vi "SPI Config Pane.vi"(6 "_SubPanelMessages":refnum<notifier>, 9 "_myEmbeddedToFrameEvent":T9, 10 "_myEmbedded.Exit":refnum<user-event>, 11 "_Property Bundle":cluster{"Name":string, "Value":variant}[](array[cluster])) -> (1 "_Connection Informations":T1, 2 "_Scripter Input":T11)   [LabVIEW 2021]
doc: "Writes data to or reads data from a serial peripheral interface (SPI) slave device."
uses:
  <vilib>/myRIO/Common/Express VI Framework/xctls/myRIO Channel Name/myRIO Channel Name.xctl
  <vilib>/myRIO/Common/Instrument Driver Framework/myRIO v1.0/SPI/typedefs/SPI Frame Length.ctl
  <vilib>/myRIO/Common/Instrument Driver Framework/myRIO v1.0/SPI/typedefs/SPI Clock Phase.ctl
  <vilib>/myRIO/Common/Instrument Driver Framework/myRIO v1.0/SPI/typedefs/SPI Clock Polarity.ctl
  <vilib>/myRIO/Common/Instrument Driver Framework/myRIO v1.0/SPI/typedefs/SPI Data Direction.ctl
  <vilib>/myRIO/Common/Express VI Framework/typedefs/Config Pane to Framework Ref.ctl
  <vilib>/myRIO/Common/Express VI Framework/typedefs/Data Validate Ref.ctl
  <vilib>/myRIO/Common/Express VI Framework/typedefs/Scripter Input.ctl
  <vilib>/myRIO/Common/Express VI Framework/typedefs/WireThrough Terminal Names.ctl
  <vilib>/myRIO/Common/Express VI Framework/typedefs/Instrument Driver Method Descriptor Array.ctl
  <vilib>/myRIO/Common/Express VI Framework/typedefs/Instrument Driver Method Descriptor.ctl
  <vilib>/myRIO/Common/Express VI Framework/typedefs/Sub Panel Messages.ctl
  <vilib>/myRIO/Common/Express VI Framework/typedefs/Connection Informations.ctl
  <vilib>/myRIO/Common/Instrument Driver Framework/Utilities/typedefs/Channel Types.ctl
  <vilib>/myRIO/Instrument Drivers/Onboard IO/SPI/typedefs/SPI User Configuration.ctl
  <vilib>/myRIO/Common/Express VI Framework/vis/Express VI Framework Strings Global.vi
  <vilib>/myRIO/Instrument Drivers/Onboard IO/SPI/SPI.lvlib
panel:
  in  "Channel:":u16(xcontrol)
  out "_learnMoreFrequency":string="Detailed information about valid frequencies for this Express VI.\nLearn more"
  in  "_Validate":bool
  in  "Frequency":dbl=1.0 caption="Frequency:" min=0.0 max=4000000.0
  in  "Frequency Unit":enum16{"Hz", "KHz", "MHz"}(ring)=enum."MHz"
  in  "Mode":enum32{"Write", "Read", "Write/Read"}(radio) caption="Mode:"
  in  "Frame length:":T2=8 min=4 max=16
  in  "Data direction:":T3
  in  "Clock polarity:":T4
  in  "Clock phase:":T5
  out "-Channel Details:":string caption="Connections:"
  in  "_Default Alias String":string
  in  "_VI Default Name (Edit and make value default)":string="SPI"
  in  "Name:":string caption="Node name:"
  in  "_WireThrough Info (Edit and make value default)":T6={"WireThrough Top In"="SPI Ref In", "WireThrough Bottom In"="error in (no error)", "WireThrough Top Out"="SPI Ref Out", "WireThrough Bottom Out"="error out"}
  in  "_Template Array (Edit and make value default)":T7=[{"Function Name"="Smart Open", "VI Path"=path "<vilib>/myRIO/Instrument Drivers/Onboard IO/SPI/vis", "Script"=TRUE, "Inputs"=[{"name"="Channel Name", "value"=variant, "Config Pane Only"=TRUE, "Build Array"=FALSE, "Bundle Cluster"=FALSE, "Show Term"=FALSE, "alias"=[], "Required Input"=FALSE}], "Outputs"=[], "VI Class"=enum."Open", "Controls Refs[]"=[], "Inline"=FALSE}, {"Function Name"="Open", "VI Path"=path "<vilib>/myRIO/Instrument Drivers/Onboard IO/SPI/vis", "Script"=FALSE, "Inputs"=[{"name"="Channel Name", "value"=variant, "Config Pane Only"=TRUE, "Build Array"=FALSE, "Bundle Cluster"=FALSE, "Show Term"=FALSE, "alias"=[], "Required Input"=FALSE}], "Outputs"=[], "VI Class"=enum."Open", "Controls Refs[]"=[], "Inline"=FALSE}, {"Function Name"="Configure", "VI Path"=path "<vilib>/myRIO/Instrument Drivers/Onboard IO/SPI/vis", "Script"=TRUE, "Inputs"=[{"name"="SPI User Configuration", "value"=variant, "Config Pane Only"=TRUE, "Build Array"=FALSE, "Bundle Cluster"=FALSE, "Show Term"=FALSE, "alias"=[], "Required Input"=FALSE}], "Outputs"=[], "VI Class"=enum."Configure", "Controls Refs[]"=[], "Inline"=FALSE}, {"Function Name"="Write Read", "VI Path"=path "<vilib>/myRIO/Instrument Drivers/Onboard IO/SPI/vis", "Script"=FALSE, "Inputs"=[{"name"="Frames to Write", "value"=variant, "Config Pane Only"=FALSE, "Build Array"=FALSE, "Bundle Cluster"=FALSE, "Show Term"=TRUE, "alias"=[], "Required Input"=TRUE}], "Outputs"=[{"name"="Frames Read", "value"=variant, "Show Term"=TRUE, "Index Array"=FALSE, "Unbundle Cluster"=FALSE, "alias"=[]}], "VI Class"=enum."Data", "Controls Refs[]"=[], "Inline"=FALSE}, {"Function Name"="Read", "VI Path"=path "<vilib>/myRIO/Instrument Drivers/Onboard IO/SPI/vis", "Script"=FALSE, "Inputs"=[{"name"="Frame Count", "value"=variant, "Config Pane Only"=FALSE, "Build Array"=FALSE, "Bundle Cluster"=FALSE, "Show Term"=TRUE, "alias"=[], "Required Input"=TRUE}], "Outputs"=[{"name"="Frames Read", "value"=variant, "Show Term"=TRUE, "Index Array"=FALSE, "Unbundle Cluster"=FALSE, "alias"=[]}], "VI Class"=enum."Data", "Controls Refs[]"=[], "Inline"=FALSE}, {"Function Name"="Write", "VI Path"=path "<vilib>/myRIO/Instrument Drivers/Onboard IO/SPI/vis", "Script"=FALSE, "Inputs"=[{"name"="Frames to Write", "value"=variant, "Config Pane Only"=FALSE, "Build Array"=FALSE, "Bundle Cluster"=FALSE, "Show Term"=TRUE, "alias"=[], "Required Input"=TRUE}], "Outputs"=[], "VI Class"=enum."Data", "Controls Refs[]"=[], "Inline"=FALSE}, {"Function Name"="Close", "VI Path"=path "<vilib>/myRIO/Instrument Drivers/Onboard IO/SPI/vis", "Script"=FALSE, "Inputs"=[], "Outputs"=[], "VI Class"=enum."Close", "Controls Refs[]"=[], "Inline"=FALSE}]
  in  "_Test Close":bool
  # "User Visible Area"
  # "NOTE: Tab Order has been set\nfor this Front Panel.\n\nSee Edit>>Set Tabbing Order...\n\nAll controls that are not visible at \nruntime are excluded from Tabbing order\n\nTo exlude a control from context\nhelp prefix its label text with a '-'"
  # "bits"
  # "Advanced options"
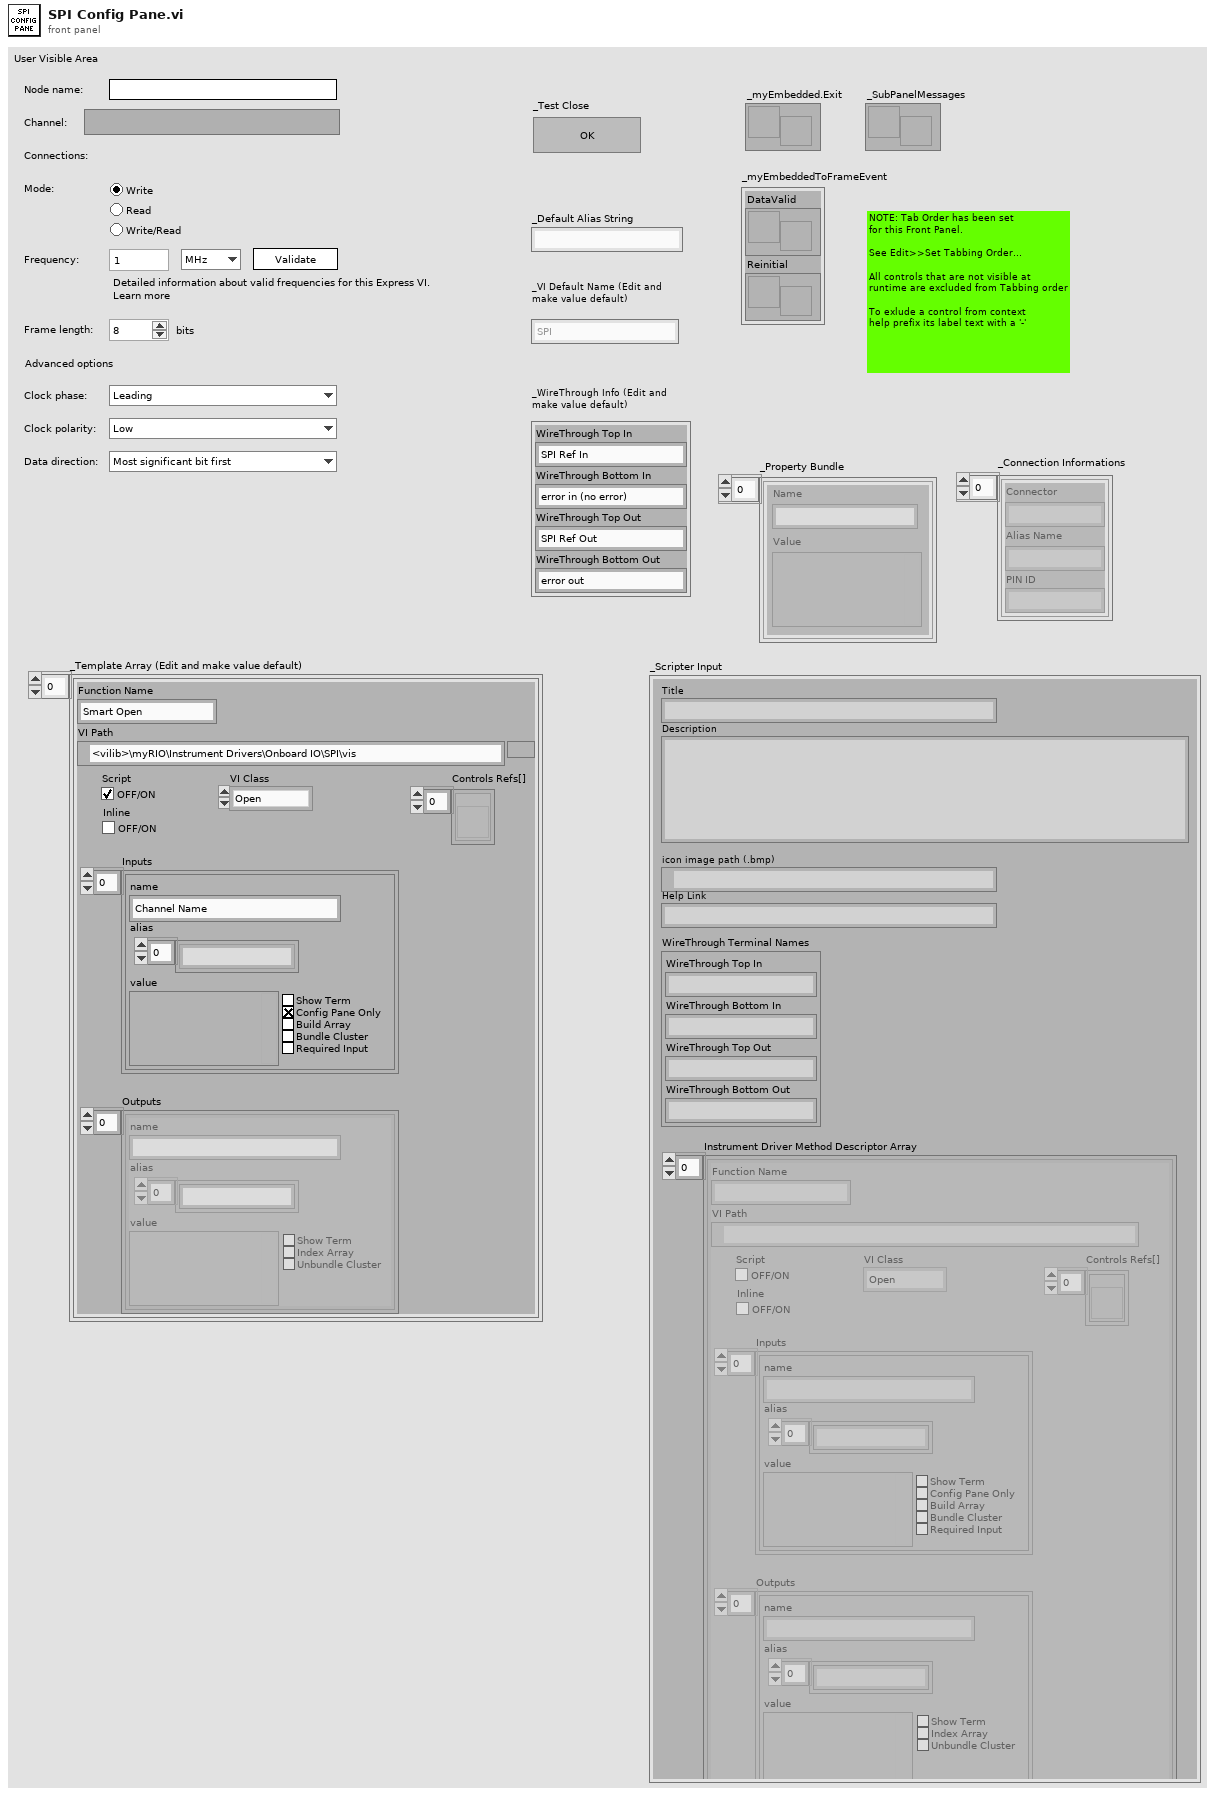
[diagram p1: front panel]
types:
  T1 = typedef "Connection Informations.ctl" = cluster{"Connector":string, "Alias Name":string, "PIN ID":string}[]
  T2 = typedef "SPI Frame Length.ctl" = u8
  T3 = typedef "SPI Data Direction.ctl" = enum8{"Most significant bit first", "Least significant bit first"}
  T4 = typedef "SPI Clock Polarity.ctl" = enum8{"Low", "High"}
  T5 = typedef "SPI Clock Phase.ctl" = enum8{"Leading", "Trailing"}
  T6 = typedef "WireThrough Terminal Names.ctl" = cluster{"WireThrough Top In":string, "WireThrough Bottom In":string, "WireThrough Top Out":string, "WireThrough Bottom Out":string}
  T7 = typedef "Instrument Driver Method Descriptor Array.ctl" = T8[]
  T8 = typedef "Instrument Driver Method Descriptor.ctl" = cluster{"Function Name":string, "VI Path":path, "Script":bool, "Inputs":cluster{"name":string, "value":variant, "Config Pane Only":bool, "Build Array":bool, "Bundle Cluster":bool, "Show Term":bool, "alias":string[], "Required Input":bool}[], "Outputs":cluster{"name":string, "value":variant, "Show Term":bool, "Index Array":bool, "Unbundle Cluster":bool, "alias":string[]}[], "VI Class":enum16{"Open", "Configure", "Data", "Manage", "Close"}, "Controls Refs[]":refnum<vi>[], "Inline":bool}
  T9 = typedef "Config Pane to Framework Ref.ctl" = cluster{"DataValid":T10, "Reinitial":refnum<user-event>}
  T10 = typedef "Data Validate Ref.ctl" = refnum<user-event>
  T11 = typedef "Scripter Input.ctl" = cluster{"Title":string, "Description":string, "icon image path (.bmp)":path, "Help Link":string, "WireThrough Terminal Names":T6, "Instrument Driver Method Descriptor Array":T7}
  T12 = typedef "Channel Types.ctl" = enum32{"Unknown", "AI", "AO", "DIO - DI", "DIO", "DIO - DO", "I2C", "PWM", "Encoder", "SPI", "UART", "Accelerometer", "DIO - LED", "DIO - Button", "AI (N Samples)", "AudioIn (N Samples)", "AO (N Samples)", "AudioOut (N Samples)", "DI (N Samples)", "DO (N Samples)", "AI IRQ", "DI IRQ", "Timer IRQ", "RSL", "Relay", "CAN", "AI (Continuous)", "AO (Continuous)"}
  T13 = typedef "Channel Info.ctl" = cluster{"Channel Name":string, "Alias":string, "Used?":bool, "Not Support?":bool, "Property Bundle":cluster{"Name":string, "Value":variant}[]}
  T14 = typedef "Sub Panel Messages.ctl" = enum16{"Initialized"}
  T15 = enum8{"Enabled", "Disabled", "Disabled and Grayed Out"}
  T16 = cluster{"Connector":string, "Alias Name":string, "PIN ID":string}
  T17 = typedef "SPI.lvlib/SPI User Configuration.ctl" = cluster{"Frequency [Hz]":dbl, "Clock Phase":T5, "Clock Polarity":T4, "Data Direction":T3, "Frame Length":T2}
  T18 = cluster{"name":string, "value":variant, "Config Pane Only":bool, "Build Array":bool, "Bundle Cluster":bool, "Show Term":bool, "alias":string[], "Required Input":bool}[]
  T19 = cluster{"name":string, "value":variant, "Config Pane Only":bool, "Build Array":bool, "Bundle Cluster":bool, "Show Term":bool, "alias":string[], "Required Input":bool}
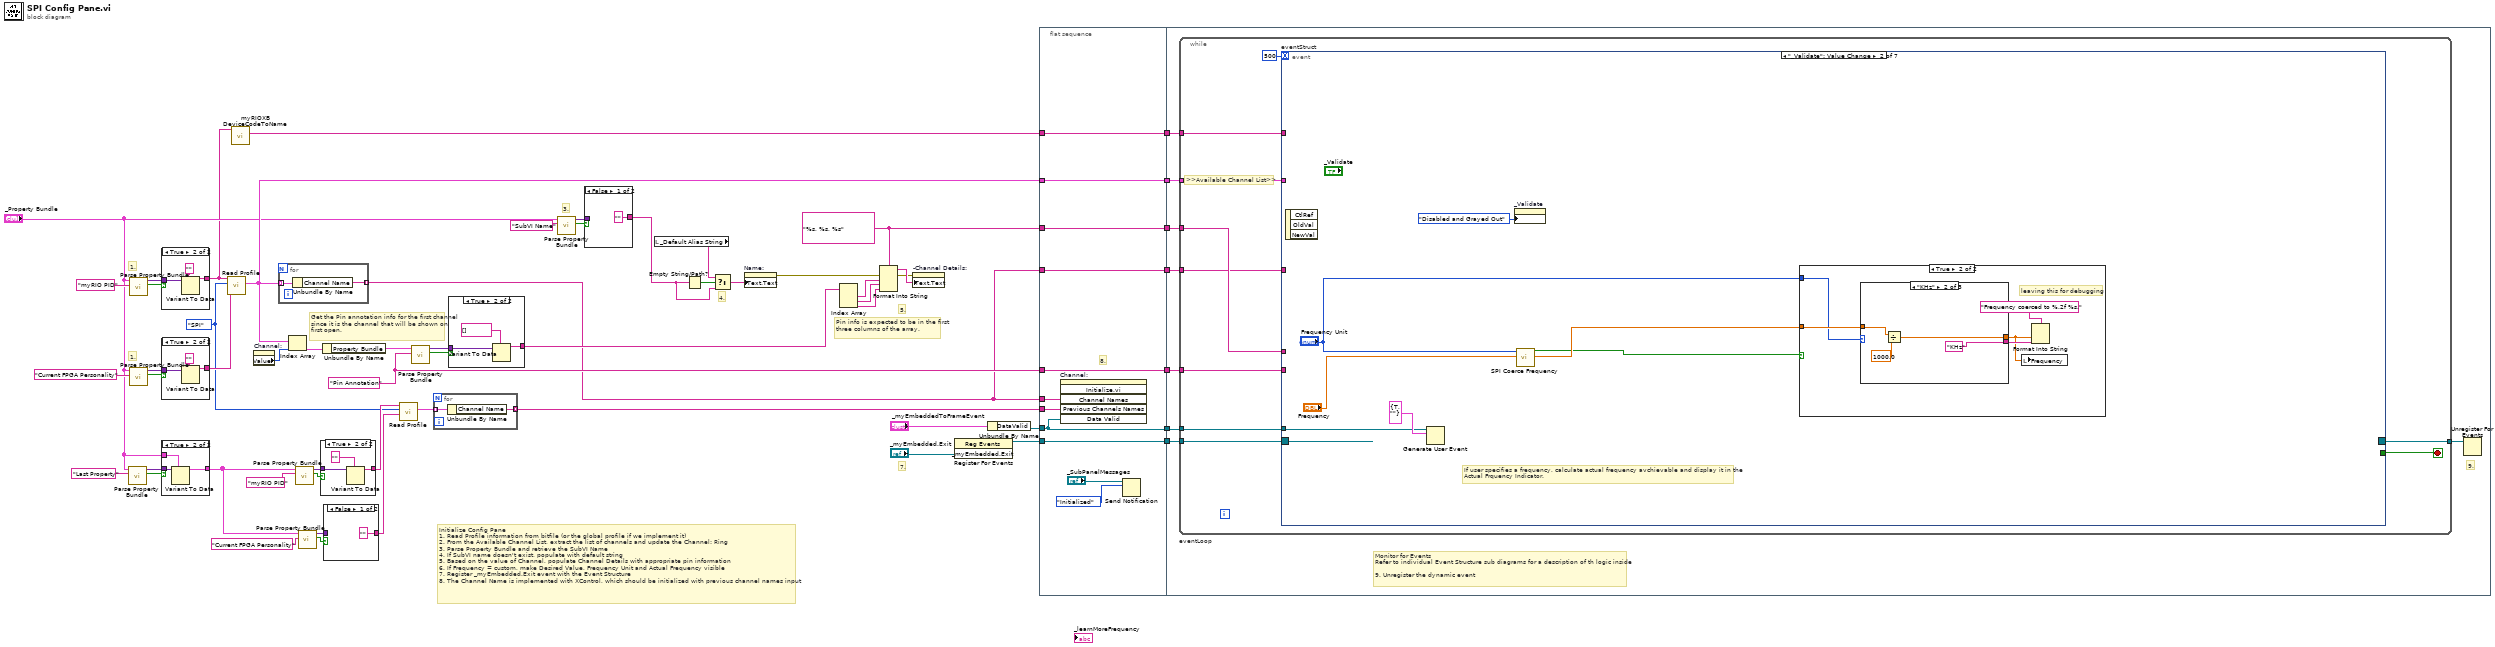
[diagram p0: block diagram]
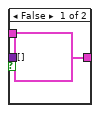
[diagram p2: hidden frame]
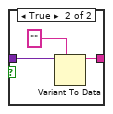
[diagram p3: hidden frame]
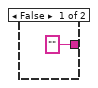
[diagram p4: hidden frame]
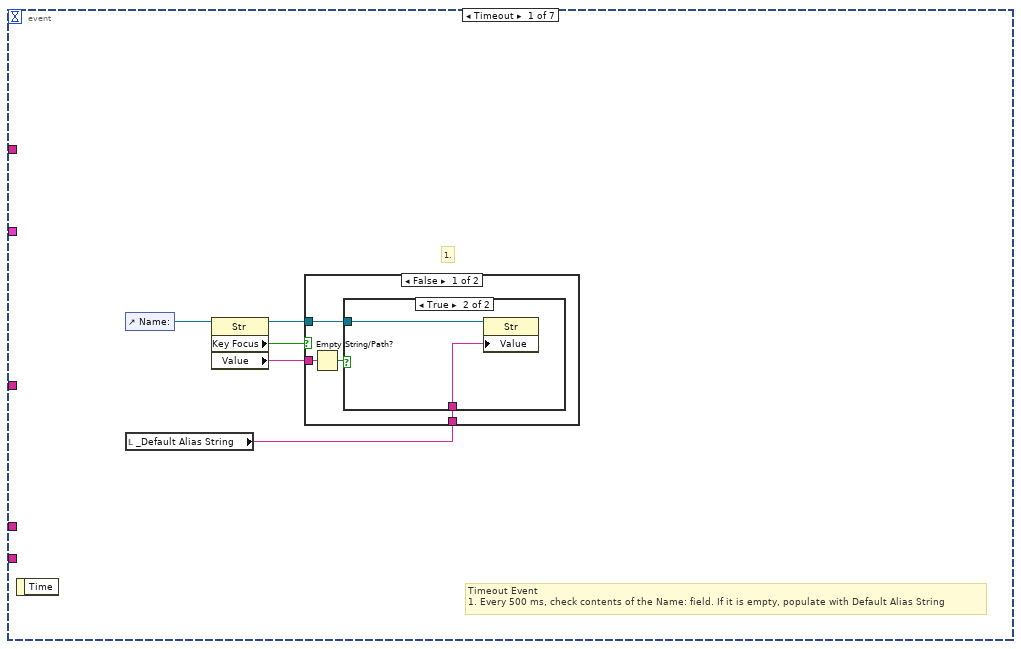
[diagram p5: hidden frame]
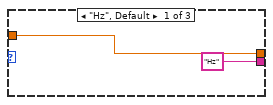
[diagram p9: hidden frame]
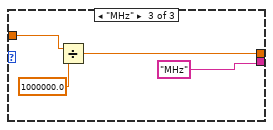
[diagram p10: hidden frame]
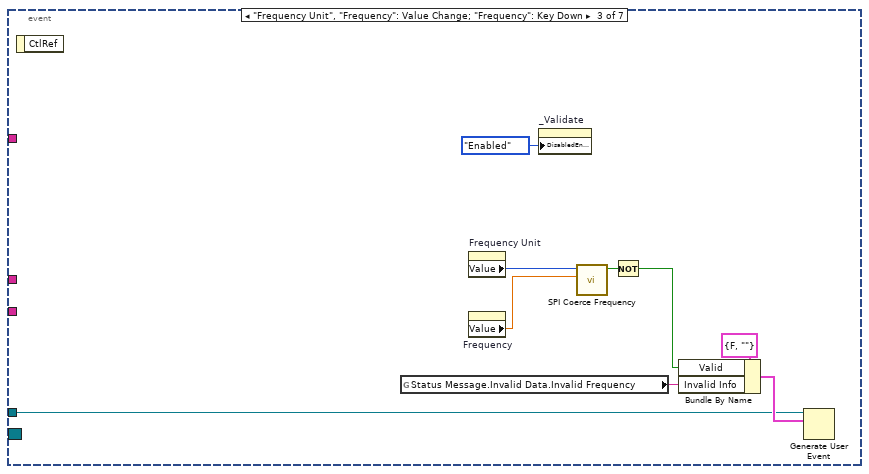
[diagram p11: hidden frame]
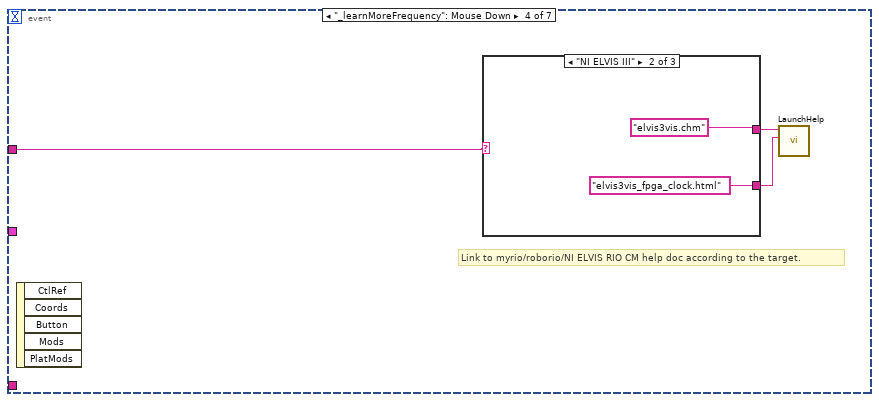
[diagram p12: hidden frame]
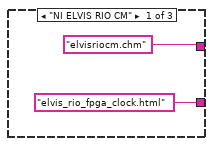
[diagram p13: hidden frame]
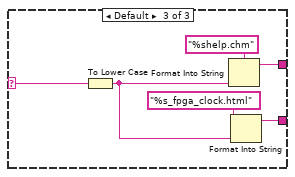
[diagram p14: hidden frame]
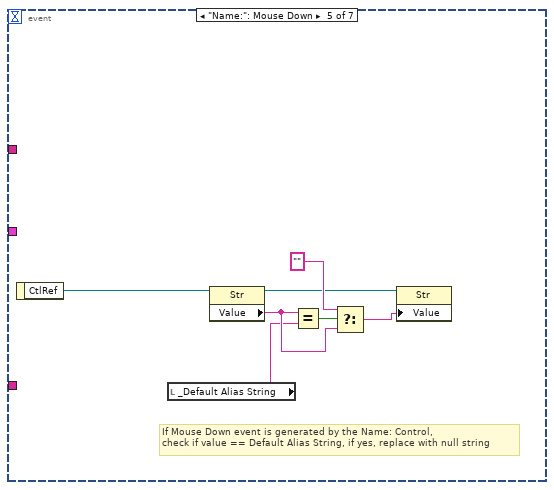
[diagram p15: hidden frame]
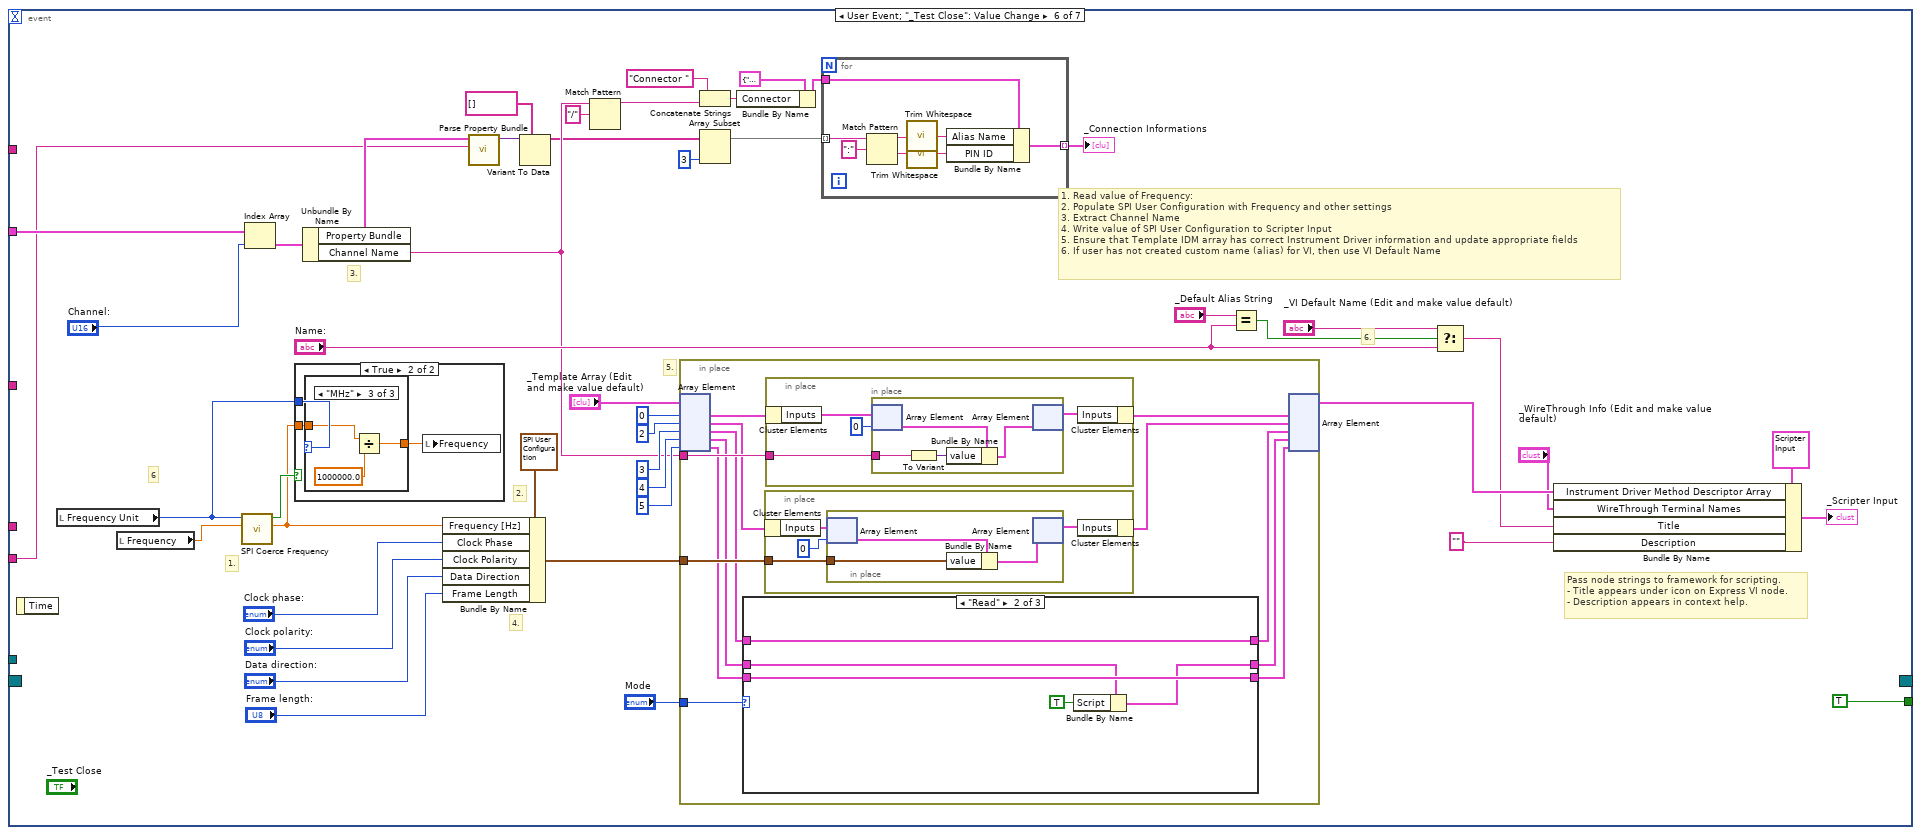
[diagram p16: hidden frame]
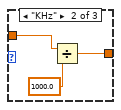
[diagram p19: hidden frame]
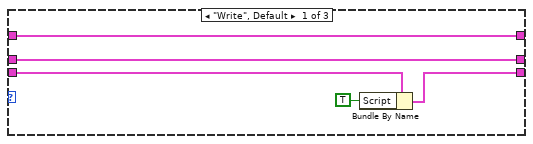
[diagram p20: hidden frame]
diagram:
  w33 = "Pin Annotation" ("Name")
  w7 = Channel_Types."SPI" ("Channel to Read")
  w43 = "%s, %s, %s"
  # "1."
  # "Pin info is expected to be in the first three columns of the array."
  # "Get the Pin annotation info for the first channel  since it is the channel that will be shown on first open."
  # "1."
  # "7."
  # "5."
  # "4."
  # "3."
  # "Initialize Config Pane\n1. Read Profile information from bitfile (or the global profile if we implement it)\n2. From the Available Channel List, extract the list of channels and update the Channel: Ring\n3. Parse Property Bundle and retrieve the SubVI Name\n4. If SubVI name doesn't exist, populate with default string\n5. Based on the value of Channel, populate Channel Details with appropriate pin information\n6. If Frequency = custom, make Desired Value, Frequency Unit and Actual Frequency visible\n7. Register _myEmbedded.Exit event with the Event Structure\n8. The Channel Name is implemented with XControl, which should be initialized with previous channel names input"
  n1 = call <vilib>:"Parse Property Bundle.vi"("Name"="Last Property", "Property Bundle"="_Property Bundle") -> ("Found?"=w11:bool, "Value"=w12:variant)  [unwired: 8 in]
  n2 = call <vilib>:"Parse Property Bundle.vi"("Name"="myRIO PID", "Property Bundle"="_Property Bundle") -> ("Found?"=w40:bool, "Value"=w41:variant)  [unwired: 8 in]
  n3 = call <vilib>:"Parse Property Bundle.vi"("Name"="Current FPGA Personality", "Property Bundle"="_Property Bundle") -> ("Found?"=w32:bool, "Value"=w31:variant)  [unwired: 8 in]
  n4 = case shown="True" w40 {
    tunnel: w41 -> [_ w63]
    tunnel: ["" ("Name") w61] -> w1
    frame False {
    }
    frame True {
      n5 = Variant To Data(type="" ("Name"), Variant=w63) -> (data=w61:string)  [unwired: 1 in, 1 out]
    }
  }
  n6 = case shown="True" w32 {
    tunnel: w31 -> [_ w67]
    tunnel: ["" ("Name") w65] -> w29
    frame False {
    }
    frame True {
      n7 = Variant To Data(type="" ("Name"), Variant=w67) -> (data=w65:string)  [unwired: 1 in, 1 out]
    }
  }
  n8 = case shown="True" w11 {
    tunnel: w12 -> [_ w71]
    tunnel: [cluster{"Name":string, "Value":variant}[] [] ("_Property Bundle") w70] -> w10
    tunnel: "_Property Bundle" -> [_ w69]
    frame False {
    }
    frame True {
      n9 = Variant To Data(type=w69, Variant=w71) -> (data=w70:cluster{"Name":string, "Value":variant}[])  [unwired: 1 in, 1 out]
    }
  }
  n10 = call <vilib>:"Read Profile.vi"("FPGA Name"=w29, "Channel to Read"=w7, "myRIO PID"=w1) -> ("Channel List Out"=w35:T13[])  [unwired: 7 in, 1 out]
  n11 = call <vilib>:"myRIOXB DeviceCodeToName.vi"("Device Code"=w1) -> ("Name"=w2:string)  [unwired: 10 in]
  n12 = property on="Channel:" class="myRIO Channel Name (strict)"() -> ("Value"=w5:u16)  [unwired: 2 in, 2 out]
  n13 = for {
    tunnel: [w73] -> w23 mode=indexing
    tunnel: w35 -> [w72] mode=indexing
    n14 = Unbundle By Name(w72) -> ("Channel Name"=w73:string)
  }
  n15 = Index Array(array=w35, index=w5) -> (element=w37:T13)
  n16 = call <vilib>:"Parse Property Bundle.vi"("Name"="myRIO PID", "Property Bundle"=w10) -> ("Found?"=w20:bool, "Value"=w19:variant)  [unwired: 8 in]
  n17 = call <vilib>:"Parse Property Bundle.vi"("Name"="Current FPGA Personality", "Property Bundle"=w10) -> ("Found?"=w15:bool, "Value"=w16:variant)  [unwired: 8 in]
  n18 = case shown="True" w20 {
    tunnel: w19 -> [_ w77]
    tunnel: ["" ("Name") w75] -> w21
    frame False {
    }
    frame True {
      n19 = Variant To Data(type="" ("Name"), Variant=w77) -> (data=w75:string)  [unwired: 1 in, 1 out]
    }
  }
  n20 = Unbundle By Name(w37) -> ("Property Bundle"=w36:cluster{"Name":string, "Value":variant}[])
  n21 = case shown="False" w15 {
    tunnel: w16 -> [_ w81]
    tunnel: ["" ("Name") w79] -> w14
    frame False {
    }
    frame True {
      n22 = Variant To Data(type="" ("Name"), Variant=w81) -> (data=w79:string)  [unwired: 1 in, 1 out]
    }
  }
  n23 = call <vilib>:"Read Profile.vi"("FPGA Name"=w14, "Channel to Read"=w7, "myRIO PID"=w21) -> ("Channel List Out"=w9:T13[])  [unwired: 7 in, 1 out]
  n24 = call <vilib>:"Parse Property Bundle.vi"("Name"=w33, "Property Bundle"=w36) -> ("Found?"=w38:bool, "Value"=w39:variant)  [unwired: 8 in]
  n25 = for {
    tunnel: [w83] -> w6 mode=indexing
    tunnel: w9 -> [w82] mode=indexing
    n26 = Unbundle By Name(w82) -> ("Channel Name"=w83:string)
  }
  n27 = case shown="True" w38 {
    tunnel: w39 -> [_ w87]
    tunnel: [string[] [] w86] -> w34
    frame False {
    }
    frame True {
      n28 = Variant To Data(type=string[] [], Variant=w87) -> (data=w86:string[])  [unwired: 1 in, 1 out]
    }
  }
  n29 = call <vilib>:"Parse Property Bundle.vi"("Name"="SubVI Name", "Property Bundle"="_Property Bundle") -> ("Found?"=w52:bool, "Value"=w51:variant)  [unwired: 8 in]
  n30 = case shown="False" w52 {
    tunnel: w51 -> [_ w91]
    tunnel: ["" ("Name") w89] -> w50
    frame False {
    }
    frame True {
      n31 = Variant To Data(type="" ("Name"), Variant=w91) -> (data=w89:string)  [unwired: 1 in, 1 out]
    }
  }
  n32 = local read "_Default Alias String"() -> (w54:string)
  n33 = Empty String/Path?(string/path=w50) -> (empty?=w56:bool)
  n34 = Select(t=w54, s=w56, f=w50) -> (s? t:f=w55:string)
  n35 = property on="Name:" class="Str"("Text.Text"=w55) -> (error out=w49:errorcluster)  [unwired: 2 in, 1 out]
  n36 = Index Array(array=w34) -> (element #1=w46:string, element #2=w45:string, element #3=w44:string)  [unwired: 3 in]
  n37 = Format Into String(format string=w43, error in=w49, w46, w45, w44) -> (resulting string=w48:string, error out=w47:errorcluster)  [unwired: 1 in]
  n38 = property on="-Channel Details:" class="Str"(error in=w47, "Text.Text"=w48) -> ()  [unwired: 1 in, 2 out]
  n39 = register-events("_myEmbedded.Exit") -> (reference out=w59:refnum<event-registration>)  [unwired: 2 in, 1 out]
  n40 = Unbundle By Name("_myEmbeddedToFrameEvent") -> ("DataValid"=w28:T10)
  n41 = flat-sequence {
    tunnel: w28 -> [w92]
    tunnel: w33 -> [w99]
    tunnel: w35 -> [w100]
    tunnel: w43 -> [w101]
    tunnel: w59 -> [w102]
    tunnel: [w102] -> w27
    tunnel: [w101] -> w26
    tunnel: [w100] -> w25
    tunnel: [w99] -> w24
    tunnel: w23 -> [w96]
    tunnel: w6 -> [w95]
    tunnel: w23 -> [w94]
    tunnel: [w94] -> w22
    tunnel: [w93] -> w4
    tunnel: w2 -> [w93]
    tunnel: [w92] -> w3
    tunnel: w27 -> [w110]
    tunnel: w26 -> [w108]
    tunnel: w25 -> [w107]
    tunnel: w24 -> [w106]
    tunnel: w22 -> [w105]
    tunnel: w4 -> [w104]
    tunnel: w3 -> [w103]
    frame #0 {
      # "8."
      n42 = invoke on="Channel:" class="myRIO Channel Name (strict)" method="Initialize.vi"("Channel Names"=w96, "Previous Channels Names"=w95, "Data Valid"=w92) -> ()  [unwired: 3 in, 6 out]
      n43 = Send Notification(notification=Sub_Panel_Messages."Initialized", notifier="_SubPanelMessages") -> ()  [unwired: 1 in, 2 out]
    }
    frame #1 {
      # "9."
      # "Monitor for Events\nRefer to individual Event Structure sub diagrams for a description of th logic inside\n\n9. Unregister the dynamic event"
      n44 = while "eventLoop" {
        tunnel: w110 -> [w119]
        tunnel: [w118] -> w109
        tunnel: w107 -> [w116]
        tunnel: w108 -> [w115]
        tunnel: w106 -> [w114]
        tunnel: w105 -> [w113]
        tunnel: w104 -> [w112]
        tunnel: w103 -> [w111]
        stop <- w120 stop-if-true
        # ">>Available Channel List>>"
        n45 = event "eventStruct" shown="[1] \"_Validate\": Value Change" {
          selector: w119 -> [_ _ _ _ _ _ _]
          dyn-events: [_ _ _ _ _ _ _] -> w118
          timeout: 500 -> [_ _ _ _ _ _ _]
          tunnel: [_ _ _ _ _ TRUE ("_Test Close") _] -> w120
          tunnel: w116 -> [_ _ _ _ _ w227 w305]
          tunnel: w115 -> [_ _ _ _ _ _ w310]
          tunnel: w114 -> [_ _ _ _ _ w187 w304]
          tunnel: w113 -> [_ _ _ _ _ _ w298]
          tunnel: w112 -> [_ _ _ w163 _ _ _]
          tunnel: w111 -> [_ w132 w157 _ _ _ w290]
          event Timeout {
            # "Timeout Event\n1. Every 500 ms, check contents of the Name: field. If it is empty, populate with Default Alias String"
            # "1."
            n46 = event-data() -> ()  [unwired: 1 in, 1 out]
            n47 = control-ref of="Name:"() -> (w123:refnum<vi>)
            n48 = local read "_Default Alias String"() -> (w121:string)
            n49 = property on="Property Node" class="Str"(reference=w123) -> (reference out=w122:refnum<vi>, "Key Focus"=w124:bool, "Value"=w125:string)  [unwired: 1 in, 1 out]
            n50 = case shown="False" w124 {
              tunnel: w125 -> [w129 _]
              tunnel: w122 -> [w127 _]
              tunnel: w121 -> [w126 _]
              frame False {
                n51 = Empty String/Path?(string/path=w129) -> (empty?=w128:bool)
                n52 = case shown="True" w128 {
                  tunnel: w127 -> [_ w131]
                  tunnel: w126 -> [_ w130]
                  frame False {
                  }
                  frame True {
                    n53 = property on="Property Node" class="Str"(reference=w131, "Value"=w130) -> ()  [unwired: 1 in, 2 out]
                  }
                }
              }
              frame True {
              }
            }
          }
          event "_Validate": Value Change {
            # "If user specifies a frequency, calculate actual frequency avchievable and display it in the \nActual Frquency Indicator."
            n54 = event-data() -> ()  [unwired: 1 in, 3 out]
            n55 = Generate User Event(user event=w132, event data cluster=cluster{"Valid":bool, "Invalid Info":string} {"Valid"=TRUE, "Invalid Info"=""} ("event data")) -> ()  [unwired: 2 in, 2 out]
            n56 = property on="_Validate" class="Bool"("DisabledEnum"=T15."Disabled and Grayed Out" ("Disabled")) -> ()  [unwired: 2 in, 2 out]
            n57 = call <vilib>:"SPI Coerce Frequency.vi"("Frequency"="Frequency", "Frequency Unit"="Frequency Unit") -> ("Actual Frequency (Hz)"=w135:dbl, "Coerced Frequency?"=w134:bool)  [unwired: 8 in]
            n58 = case shown="True" w134 {
              tunnel: w135 -> [_ w143]
              tunnel: "Frequency Unit" -> [_ w140]
              frame False {
              }
              frame True {
                # "leaving this for debugging"
                n59 = case shown="\"KHz\"" w140 {
                  tunnel: w143 -> [w145 w149 w152]
                  tunnel: [w145 w148 w150] -> w139
                  tunnel: ["Hz" ("format string") "KHz" ("format string") "MHz" ("format string")] -> w141
                  frame "Hz", Default {
                  }
                  frame "KHz" {
                    n60 = Divide(x=w149, y=1000.0) -> (x/y=w148:dbl)
                  }
                  frame "MHz" {
                    n61 = Divide(x=w152, y=1000000.0) -> (x/y=w150:dbl)
                  }
                }
                n62 = local write "Frequency"(w139) -> ()
                n63 = Format Into String(format string="Frequency coerced to %.2f %s.", w139, w141) -> ()  [unwired: 2 in, 2 out]
              }
            }
          }
          event "Frequency Unit", "Frequency": Value Change; "Frequency": Key Down {
            n64 = event-data() -> ()  [unwired: 1 in, 1 out]
            n65 = global read "Express VI Framework Strings Global.vi" "Status Message.Invalid Data.Invalid Frequency"() -> (w158:string)
            n66 = property on="Frequency Unit" class="Enum (strict)"() -> ("Value"=w156:enum16{"Hz", "KHz", "MHz"})  [unwired: 2 in, 2 out]
            n67 = property on="Frequency" class="DigNum (strict)"() -> ("Value"=w155:dbl)  [unwired: 2 in, 2 out]
            n68 = property on="_Validate" class="Bool"("DisabledEnum"=T15."Enabled" ("Disabled")) -> ()  [unwired: 2 in, 2 out]
            n69 = call <vilib>:"SPI Coerce Frequency.vi"("Frequency"=w155, "Frequency Unit"=w156) -> ("Coerced Frequency?"=w154:bool)  [unwired: 8 in, 1 out]
            n70 = Not(x=w154) -> (.not. x?=w159:bool)
            n71 = Bundle By Name(cluster=cluster{"Valid":bool, "Invalid Info":string} {"Valid"=FALSE, "Invalid Info"=""} ("event data"), "Valid"=w159, "Invalid Info"=w158) -> (w160:cluster{"Valid":bool, "Invalid Info":string})
            n72 = Generate User Event(user event=w157, event data cluster=w160) -> ()  [unwired: 2 in, 2 out]
          }
          event "_learnMoreFrequency": Mouse Down {
            # "Link to myrio/roborio/NI ELVIS RIO CM help doc according to the target."
            n73 = event-data() -> ()  [unwired: 1 in, 5 out]
            n74 = case shown="\"NI ELVIS III\"" w163 {
              selector: w163 -> [_ _ w170]
              tunnel: ["elvisriocm.chm" ("Help File") "elvis3vis.chm" ("Help File") w172] -> w165
              tunnel: ["elvis_rio_fpga_clock.html" ("Help Topic") "elvis3vis_fpga_clock.html" ("Help Topic") w171] -> w164
              frame "NI ELVIS RIO CM" {
              }
              frame "NI ELVIS III" {
              }
              frame Default {
                n75 = To Lower Case(string=w170) -> (all lower case string=w174:string)
                n76 = Format Into String(format string="%shelp.chm" ("Help File"), w174) -> (resulting string=w172:string)  [unwired: 2 in, 1 out]
                n77 = Format Into String(format string="%s_fpga_clock.html" ("Help Topic"), w174) -> (resulting string=w171:string)  [unwired: 2 in, 1 out]
              }
            }
            n78 = call <vilib>:"LaunchHelp.vi"("Help Topic"=w164, "Help File"=w165) -> ()  [unwired: 10 in]
          }
          event "Name:": Mouse Down {
            # "If Mouse Down event is generated by the Name: Control,\ncheck if value == Default Alias String, if yes, replace with null string"
            n79 = event-data() -> ("CtlRef"=w182:refnum<vi>)  [unwired: 1 in]
            n80 = local read "_Default Alias String"() -> (w176:string)
            n81 = property class="Str"(reference=w182) -> (reference out=w178:refnum<vi>, "Value"=w177:string)  [unwired: 1 in, 1 out]
            n82 = Equal?(x=w177, y=w176) -> (x = y?=w181:bool)
            n83 = Select(t="", s=w181, f=w177) -> (s? t:f=w179:string)
            n84 = property class="Str"(reference=w178, "Value"=w179) -> ()  [unwired: 1 in, 2 out]
          }
          event User Event; "_Test Close": Value Change {
            # "6"
            # "3."
            # "4."
            # "2."
            # "1. Read value of Frequency:\n2. Populate SPI User Configuration with Frequency and other settings\n3. Extract Channel Name\n4. Write value of SPI User Configuration to Scripter Input\n5. Ensure that Template IDM array has correct Instrument Driver information and update appropriate fields\n6. If user has not created custom name (alias) for VI, then use VI Default Name"
            # "6."
            # "5."
            # "1."
            # "Pass node strings to framework for scripting.\n- Title appears under icon on Express VI node.\n- Description appears in context help."
            n85 = event-data() -> ()  [unwired: 1 in, 1 out]
            n86 = local read "Frequency Unit"() -> (w201:enum16{"Hz", "KHz", "MHz"})
            n87 = local read "Frequency"() -> (w202:dbl)
            n88 = call <vilib>:"SPI Coerce Frequency.vi"("Frequency"=w202, "Frequency Unit"=w201) -> ("Actual Frequency (Hz)"=w199:dbl, "Coerced Frequency?"=w200:bool)  [unwired: 8 in]
            n89 = Index Array(array=w227, index="Channel:") -> (element=w207:T13)
            n90 = case shown="True" w200 {
              tunnel: w199 -> [_ w239]
              tunnel: w201 -> [_ w238]
              frame False {
              }
              frame True {
                n91 = case shown="\"MHz\"" w238 {
                  tunnel: w239 -> [w240 w243 w245]
                  tunnel: [w240 w242 w244] -> w237
                  frame "Hz", Default {
                  }
                  frame "KHz" {
                    n92 = Divide(x=w243, y=1000.0) -> (x/y=w242:dbl)
                  }
                  frame "MHz" {
                    n93 = Divide(x=w245, y=1000000.0) -> (x/y=w244:dbl)
                  }
                }
                n94 = local write "Frequency"(w237) -> ()
              }
            }
            n95 = Unbundle By Name(w207) -> ("Property Bundle"=w188:cluster{"Name":string, "Value":variant}[], "Channel Name"=w190:string)
            n96 = Bundle By Name(cluster=T17 {"Frequency [Hz]"=0.0, "Clock Phase"=enum."Leading", "Clock Polarity"=enum."Low", "Data Direction"=enum."Most significant bit first", "Frame Length"=8} ("SPI User Configuration"), "Frequency [Hz]"=w199, "Clock Phase"="Clock phase:", "Clock Polarity"="Clock polarity:", "Data Direction"="Data direction:", "Frame Length"="Frame length:") -> (w214:T17)
            n97 = call <vilib>:"Parse Property Bundle.vi"("Name"=w187, "Property Bundle"=w188) -> ("Value"=w191:variant)  [unwired: 8 in, 1 out]
            n98 = Variant To Data(type=string[] [], Variant=w191) -> (data=w185:string[])  [unwired: 1 in, 1 out]
            n99 = Match Pattern(string=w190, regular expression="/") -> (before substring=w196:string)  [unwired: 1 in, 3 out]
            n100 = in-place {
              in-place-border: w190 -> [w257]
              in-place-border: w214 -> [w254]
              in-place-border: "Mode" -> [w253]
              n101 = in-place-array #1("_Template Array (Edit and make value default)", 0, 2, 3, 4, 5) -> (w259:T8, w256:T8, w252:T8, w250:T8, w247:T8)
              n102 = case shown="\"Read\"" w253 {
                tunnel: w252 -> [w264 w268 w273]
                tunnel: [w264 w268 w272] -> w251
                tunnel: w250 -> [w263 w267 w274]
                tunnel: [w263 w266 w274] -> w249
                tunnel: [w261 w269 w270] -> w248
                tunnel: w247 -> [w262 w269 w270]
                frame "Write", Default {
                  n103 = Bundle By Name(cluster=w262, "Script"=TRUE) -> (w261:T8)
                }
                frame "Read" {
                  n104 = Bundle By Name(cluster=w267, "Script"=TRUE) -> (w266:T8)
                }
                frame "Write/Read" {
                  n105 = Bundle By Name(cluster=w273, "Script"=TRUE) -> (w272:T8)
                }
              }
              n106 = in-place {
                in-place-border: w254 -> [w275]
                n107 = in-place-cluster #2(w256) -> ("Inputs"=w278:T18)
                n108 = in-place {
                  in-place-border: w275 -> [w279]
                  n109 = in-place-array #3(w278, 0) -> (w281:T19)
                  n110 = Bundle By Name(cluster=w281, "value"=w279) -> (w280:T19)
                  n111 = in-place-array #3(w280) -> (w277:T18)  [unwired: 1 out]
                }
                n112 = in-place-cluster #2("Inputs"=w277) -> (w255:T8)
              }
              n113 = in-place {
                in-place-border: w257 -> [w284]
                n114 = in-place-cluster #4(w259) -> ("Inputs"=w285:T18)
                n115 = in-place {
                  in-place-border: w284 -> [w286]
                  n116 = in-place-array #5(w285, 0) -> (w289:T19)
                  n117 = To Variant(anything=w286) -> (Variant=w287:variant)
                  n118 = Bundle By Name(cluster=w289, "value"=w287) -> (w288:T19)
                  n119 = in-place-array #5(w288) -> (w283:T18)  [unwired: 1 out]
                }
                n120 = in-place-cluster #4("Inputs"=w283) -> (w258:T8)
              }
              n121 = in-place-array #1(w258, w255, w251, w249, w248) -> (w225:T7)  [unwired: 5 out]
            }
            n122 = Concatenate Strings("Connector " ("string"), w196) -> (w198:string)
            n123 = Array Subset(array=w185, length=3) -> (w186:string[])  [unwired: 1 in]
            n124 = Bundle By Name(cluster=T16 {"Connector"="", "Alias Name"="", "PIN ID"=""} ("Connection Information"), "Connector"=w198) -> (w194:T16)
            n125 = for {
              tunnel: w186 -> [w235] mode=indexing
              tunnel: w194 -> [w236]
              tunnel: [w231] -> w189 mode=indexing
              n126 = Match Pattern(string=w235, regular expression=":") -> (before substring=w233:string, after substring=w232:string)  [unwired: 1 in, 2 out]
              n127 = call <vilib>:"Trim Whitespace.vi"("string"=w233) -> ("trimmed string"=w230:string)  [unwired: 1 in]
              n128 = call <vilib>:"Trim Whitespace.vi"("string"=w232) -> ("trimmed string"=w229:string)  [unwired: 1 in]
              n129 = Bundle By Name(cluster=w236, "Alias Name"=w230, "PIN ID"=w229) -> (w231:T16)
            }
            "_Connection Informations" <- w189
            n130 = Equal?(x="_Default Alias String", y="Name:") -> (x = y?=w217:bool)
            n131 = Select(t="_VI Default Name (Edit and make value default)", s=w217, f="Name:") -> (s? t:f=w216:string)
            n132 = Bundle By Name(cluster=T11 {"Title"="", "Description"="", "icon image path (.bmp)"=path "", "Help Link"="", "WireThrough Terminal Names"={"WireThrough Top In"="", "WireThrough Bottom In"="", "WireThrough Top Out"="", "WireThrough Bottom Out"=""}, "Instrument Driver Method Descriptor Array"=[]} ("Scripter Input"), "Instrument Driver Method Descriptor Array"=w225, "WireThrough Terminal Names"="_WireThrough Info (Edit and make value default)", "Title"=w216, "Description"="" ("Title")) -> (→"_Scripter Input":T11)
          }
          event "Channel:": Value Change {
            # "1."
            # "1. When Channel changes, check if Name: matches any of the channels in the Channel list. \nIf so, you replace Name: with the default string\n2. Look up pin information for Channel and populate Channel Details."
            # "2."
            n133 = event-data() -> ()  [unwired: 1 in, 1 out]
            n134 = property on="Name:" class="Str"() -> ("Text.Text"=w314:string)  [unwired: 2 in, 2 out]
            n135 = property on="Channel:" class="myRIO Channel Name (strict)"() -> ("Value"=w299:u16)  [unwired: 2 in, 2 out]
            n136 = local read "_Default Alias String"() -> (w312:string)
            n137 = Index Array(array=w305, index=w299) -> (element=w308:T13)
            n138 = Search 1D Array(1D array=w298, element=w314) -> (index of element=w317:i32)  [unwired: 1 in]
            n139 = Unbundle By Name(w308) -> ("Property Bundle"=w309:cluster{"Name":string, "Value":variant}[])
            n140 = Not Equal?(x=w317, y=-1) -> (x != y?=w315:bool)
            n141 = Select(t=w312, s=w315, f=w314) -> (s? t:f=w313:string)
            n142 = property on="Name:" class="Str"("Text.Text"=w313) -> ()  [unwired: 2 in, 2 out]
            n143 = call <vilib>:"Parse Property Bundle.vi"("Name"=w304, "Property Bundle"=w309) -> ("Found?"=w307:bool, "Value"=w306:variant)  [unwired: 8 in]
            n144 = case shown="True" w307 {
              tunnel: w306 -> [_ w321]
              tunnel: [string[] [] w320] -> w303
              frame False {
              }
              frame True {
                n145 = Variant To Data(type=string[] [], Variant=w321) -> (data=w320:string[])  [unwired: 1 in, 1 out]
              }
            }
            n146 = Index Array(array=w303) -> (element #1=w302:string, element #2=w301:string, element #3=w300:string)  [unwired: 3 in]
            n147 = Format Into String(format string=w310, w302, w301, w300) -> (resulting string=→"-Channel Details:":string)  [unwired: 2 in, 1 out]
            n148 = global read "Express VI Framework Strings Global.vi" "Status Message.Invalid Data.Invalid Frequency"() -> (w294:string)
            n149 = property on="Frequency Unit" class="Enum (strict)"() -> ("Value"=w293:enum16{"Hz", "KHz", "MHz"})  [unwired: 2 in, 2 out]
            n150 = property on="Frequency" class="DigNum (strict)"() -> ("Value"=w292:dbl)  [unwired: 2 in, 2 out]
            n151 = call <vilib>:"SPI Coerce Frequency.vi"("Frequency"=w292, "Frequency Unit"=w293) -> ("Coerced Frequency?"=w291:bool)  [unwired: 8 in, 1 out]
            n152 = Not(x=w291) -> (.not. x?=w295:bool)
            n153 = Bundle By Name(cluster=cluster{"Valid":bool, "Invalid Info":string} {"Valid"=FALSE, "Invalid Info"=""} ("event data"), "Valid"=w295, "Invalid Info"=w294) -> (w296:cluster{"Valid":bool, "Invalid Info":string})
            n154 = Generate User Event(user event=w290, event data cluster=w296) -> ()  [unwired: 2 in, 2 out]
          }
        }
      }
      n155 = Unregister For Events(event registration refnum=w109) -> ()  [unwired: 1 in, 1 out]
    }
  }
